vi "test variant to json string.vi"(8 "error in (no error)":errorcluster) -> (0 "error out":errorcluster)   [LabVIEW 2019, in "labview_json_tests.lvlib"]
uses:
  labview_json_tests.lvlib
  lib/labview_json.lvlib
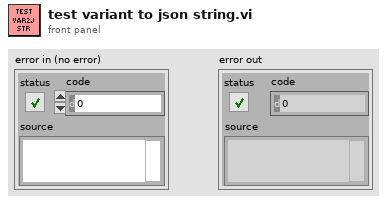
[diagram p1: front panel]
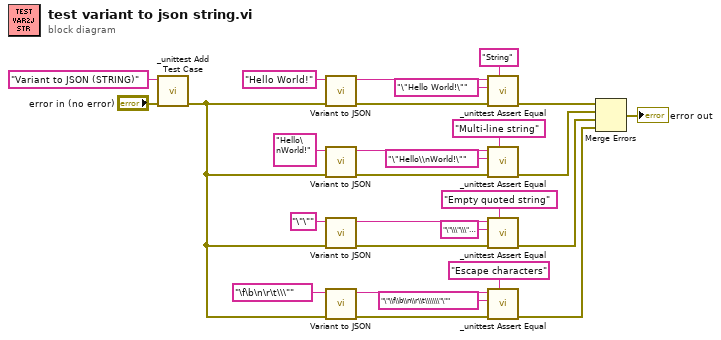
[diagram p0: block diagram]
diagram:
  n1 = call "_unittest Add Test Case.vi"("error in (no error)"="error in (no error)", "Test Case"="Variant to JSON (STRING)") -> ("error out"=w1:errorcluster)  [unwired: 9 in]
  n2 = call "Variant to JSON.vi"("error in (no error)"=w1, "Variant in"="Hello World!") -> ("error out"=w21:errorcluster, "JSON"=w20:string)  [unwired: 8 in]
  n3 = call "Variant to JSON.vi"("error in (no error)"=w1, "Variant in"="Hello\nWorld!") -> ("error out"=w19:errorcluster, "JSON"=w18:string)  [unwired: 8 in]
  n4 = call "Variant to JSON.vi"("error in (no error)"=w1, "Variant in"="\"\"") -> ("error out"=w10:errorcluster, "JSON"=w11:string)  [unwired: 8 in]
  n5 = call "Variant to JSON.vi"("error in (no error)"=w1, "Variant in"="\f\b\n\r\t\\\"") -> ("error out"=w12:errorcluster, "JSON"=w13:string)  [unwired: 8 in]
  n6 = call "_unittest Assert Equal.vi"("Message"="String", "error in (no error)"=w21, "Expected Value"="\"Hello World!\"", "Actual Value"=w20) -> ("error out"=w26:errorcluster)  [unwired: 7 in]
  n7 = call "_unittest Assert Equal.vi"("Message"="Multi-line string", "error in (no error)"=w19, "Expected Value"="\"Hello\\nWorld!\"", "Actual Value"=w18) -> ("error out"=w22:errorcluster)  [unwired: 7 in]
  n8 = call "_unittest Assert Equal.vi"("Message"="Empty quoted string", "error in (no error)"=w10, "Expected Value"="\"\\\"\\\"\"", "Actual Value"=w11) -> ("error out"=w7:errorcluster)  [unwired: 7 in]
  n9 = call "_unittest Assert Equal.vi"("Message"="Escape characters", "error in (no error)"=w12, "Expected Value"="\"\\f\\b\\n\\r\\t\\\\\\\"\"", "Actual Value"=w13) -> ("error out"=w6:errorcluster)  [unwired: 7 in]
  n10 = Merge Errors(w26, w22, w7, w6) -> (→"error out":errorcluster)
